vi "Convert HexString to String.vi"(1 "String (Hex)":string) -> (0 "String":string)   [LabVIEW 2013]
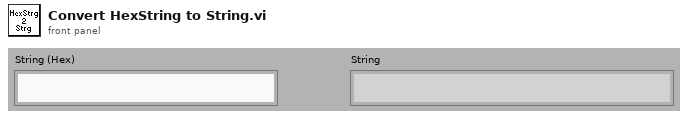
[diagram p1: front panel]
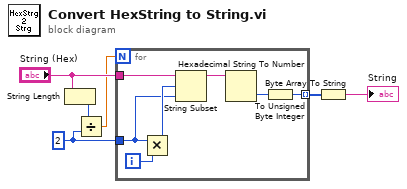
[diagram p0: block diagram]
diagram:
  w3 = 2 ("y")
  n1 = String Length(string="String (Hex)") -> (length=w5:i32)
  n2 = Divide(x=w5, y=w3) -> (x/y=w4:dbl)
  n3 = for {
    N: w4 -> [_]
    tunnel: "String (Hex)" -> [w12]
    tunnel: w3 -> [w10]
    tunnel: [w7] -> w2 mode=indexing
    i -> [w13]
    n4 = Multiply(x=w10, y=w13) -> (x*y=w11:i32)
    n5 = String Subset(string=w12, offset (0)=w11, length (rest)=w10) -> (substring=w9:string)
    n6 = Hexadecimal String To Number(string=w9) -> (number=w8:u32)  [unwired: 2 in, 1 out]
    n7 = To Unsigned Byte Integer(number=w8) -> (unsigned 8bit integer=w7:u8)
  }
  n8 = Byte Array To String(unsigned byte array=w2) -> (string=→"String":string)
